vi "SW_Generate_Full_Condition(s)_text.vi"(8 "error in (no error)":errorcluster, 9 "Array of conditions in":T1 {"Response"."TTL pulse length, ms" min=0.0 max=10000.0 step=10.0 format="%0.0g"; "Specifier(s)"."Validity criteria(s)"."Validity value" min=0.0 step=0.1 format="%.2g"; "Specifier(s)"."Value" step=1.0 format="%#.2g"}, 10 "Calibration parameters":T7 {"True frame time, s" format="%.10g"; "Disp. calibration info"."Speed, µl per ms" format="%.3g"; "True FPS" format="%.10g"; "Timing calibration sw/hw" format="%.10g"}, 11 "TreeControl in":refnum<vi>) -> (0 "error out":errorcluster)   [LabVIEW 2018, in "Tracker.lvlib"]
uses:
  Tracker.lvlib
  Controls/CTL_Calibration_parameters.ctl
  Controls/CTL_Dispenser_calibration_info.ctl
  Controls/CTL_Conditions_Array.ctl
  Controls/CTL_Conditions_Cluster.ctl
  Controls/CTL_Condition_type.ctl
  Controls/CTL_Comparison_type.ctl
  Controls/CTL_Validity_check_criteria.ctl
  Controls/CTL_Condition_response_type.ctl
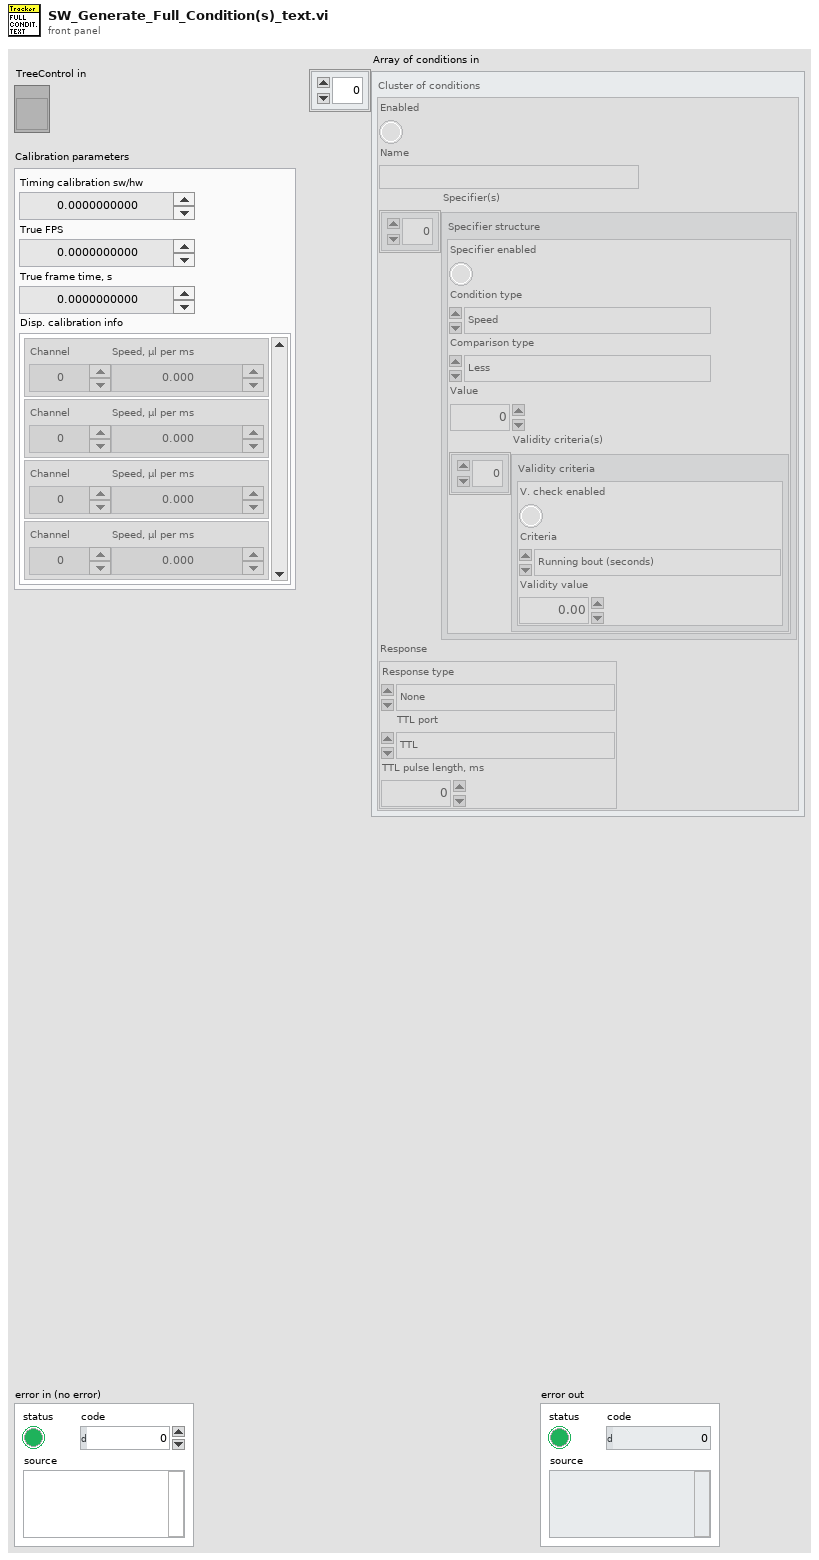
[diagram p1: front panel]
types:
  T1 = typedef "Tracker.lvlib/CTL_Conditions_Array.ctl" = T2[]
  T2 = typedef "Tracker.lvlib/CTL_Conditions_Cluster.ctl" = cluster{"Enabled":bool, "Name":string, "Specifier(s)":cluster{"Specifier enabled":bool, "Condition type":T3, "Comparison type":T4, "Value":dbl, "Validity criteria(s)":cluster{"V. check enabled":bool, "Criteria":T5, "Validity value":dbl}[]}[], "Response":cluster{"Response type":T6, "TTL port":enum16{"TTL"}, "TTL pulse length, ms":dbl}}
  T3 = typedef "Tracker.lvlib/CTL_Condition_type.ctl" = enum16{"Speed", "Zone", "Angle to wall"}
  T4 = typedef "Tracker.lvlib/CTL_Comparison_type.ctl" = enum16{"Less", "Less or Equal", "Equal", "Greater or Equal", "Greater", "Not Equal"}
  T5 = typedef "Tracker.lvlib/CTL_Validity_check_criteria.ctl" = enum16{"Running bout (seconds)", "Running bout (meters)"}
  T6 = typedef "Tracker.lvlib/CTL_Condition_response_type.ctl" = enum16{"None", "Air puff", "Liquid reward"}
  T7 = typedef "Tracker.lvlib/CTL_Calibration_parameters.ctl" = cluster{"Timing calibration sw/hw":dbl, "True FPS":dbl, "True frame time, s":dbl, "Disp. calibration info":T8}
  T8 = typedef "Tracker.lvlib/CTL_Dispenser_calibration_info.ctl" = cluster{"Channel":u8, "Speed, µl per ms":dbl}[]
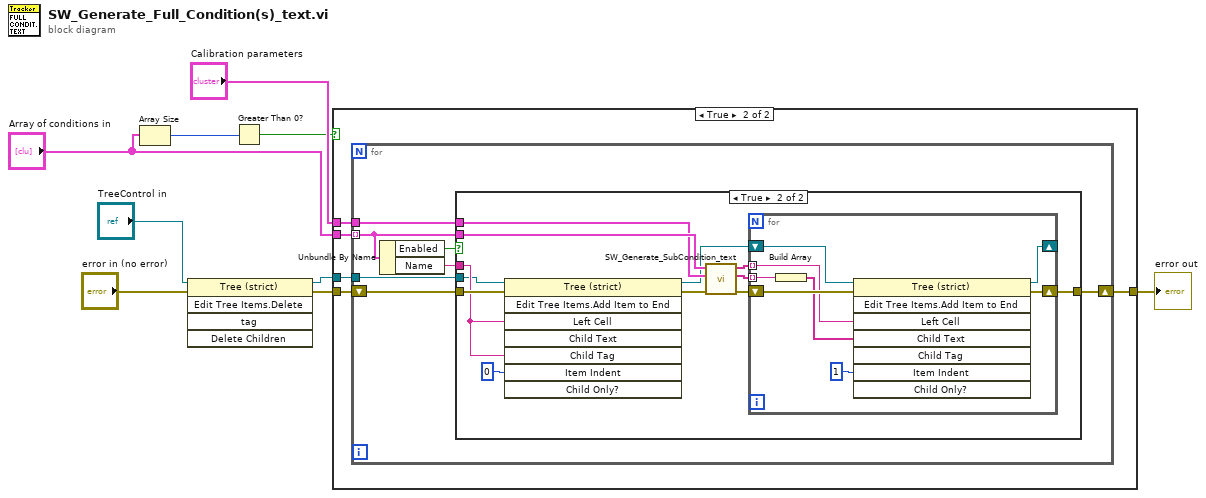
[diagram p0: block diagram]
diagram:
  n1 = Array Size(array="Array of conditions in") -> (size(s)=w7:i32)
  n2 = invoke on="Invoke Node" class="Tree (strict)" method="Edit Tree Items.Delete"(reference="TreeControl in", error in="error in (no error)") -> (reference out=w1:refnum<vi>, error out=w6:errorcluster)  [unwired: 3 in, 3 out]
  n3 = Greater Than 0?(x=w7) -> (x > 0?=w3:bool)
  n4 = case shown="True" w3 {
    tunnel: "Array of conditions in" -> [_ w15]
    tunnel: w6 -> [w10 w14]
    tunnel: [w10 w13] -> w8
    tunnel: "Calibration parameters" -> [_ w12]
    tunnel: w1 -> [_ w11]
    frame False {
    }
    frame True {
      n5 = for {
        tunnel: w15 -> [w19] mode=indexing
        shift-right: [w20] -> w13
        shift-left: w14 -> [w21]
        tunnel: w12 -> [w17]
        tunnel: w11 -> [w16]
        n6 = Unbundle By Name(w19) -> ("Enabled"=w18:bool, "Name"=w22:string)
        n7 = case shown="True" w18 {
          tunnel: w22 -> [_ w27]
          tunnel: w21 -> [w23 w35]
          tunnel: [w23 w31] -> w20
          tunnel: w19 -> [_ w30]
          tunnel: w17 -> [_ w26]
          tunnel: w16 -> [_ w25]
          frame False {
          }
          frame True {
            n8 = invoke on="Invoke Node" class="Tree (strict)" method="Edit Tree Items.Add Item to End"(reference=w25, error in=w35, "Left Cell"=w27, "Child Tag"=w27, "Item Indent"=0 ("New Item Indentation")) -> (reference out=w24:refnum<vi>, error out=w34:errorcluster)  [unwired: 3 in, 6 out]
            n9 = call "SW_Generate_SubCondition_text.vi"("error in (no error)"=w34, "Calibration parameters"=w26, "Condition"=w30) -> ("error out"=w32:errorcluster, "Validity criteria"=w28:string[], "SubCondition"=w29:string[])  [unwired: 6 in]
            n10 = for {
              shift-right: [w42] -> w31
              shift-left: w32 -> [w43]
              tunnel: w29 -> [w40] mode=indexing
              tunnel: w28 -> [w39] mode=indexing
              shift-right: [w36] -> _
              shift-left: w24 -> [w37]
              n11 = Build Array(w39) -> (w38:string[])
              n12 = invoke on="Invoke Node" class="Tree (strict)" method="Edit Tree Items.Add Item to End"(reference=w37, error in=w43, "Left Cell"=w40, "Child Text"=w38, "Item Indent"=1 ("New Item Indentation")) -> (reference out=w36:refnum<vi>, error out=w42:errorcluster)  [unwired: 3 in, 6 out]
            }
          }
        }
      }
    }
  }
  "error out" <- w8
